vi "Instrument Typecast.vi"(8 "error in (no error)":errorcluster, 11 "pin instrument":refnum<class>) -> (0 "error out":errorcluster, 3 "instrument object":refnum<class "DMM_Base.lvclass">)   [LabVIEW 2021, in "DMM_Base.lvclass"]
uses:
  DMM_Base.lvclass
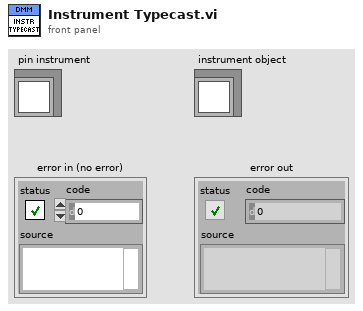
[diagram p1: front panel]
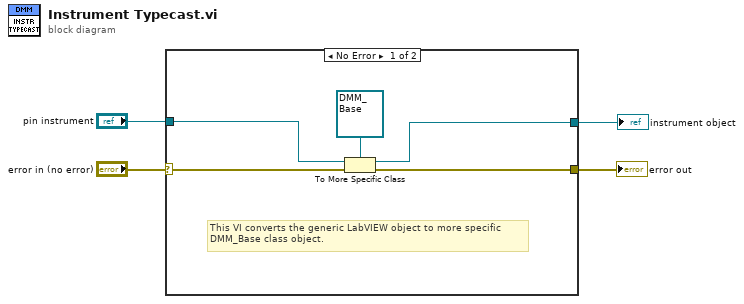
[diagram p0: block diagram]
diagram:
  n1 = case shown="No Error" "error in (no error)" {
    selector: "error in (no error)" -> [w9 w10]
    tunnel: "pin instrument" -> [w8 _]
    tunnel: [w6 w10] -> w2
    tunnel: [w5 _] -> w1
    frame No Error {
      # "This VI converts the generic LabVIEW object to more specific\nDMM_Base class object."
      n2 = To More Specific Class(target class=refnum<class "DMM_Base.lvclass"> refnum ("DMM_Base.lvclass"), reference=w8, error in=w9) -> (specific class reference=w5:refnum<class "DMM_Base.lvclass">, error out=w6:errorcluster)
    }
    frame Error {
    }
  }
  "error out" <- w2
  "instrument object" <- w1
